vi "Flatten Value.vi"(0 "Path In":refnum<class "Path.lvclass">, 11 "Error In":errorcluster) -> (4 "Path Out":refnum<class "Path.lvclass">, 8 "Value":string, 15 "Error Out":errorcluster)   [LabVIEW 2016, in "Path.lvclass"]
uses:
  Path.lvclass
  Path.lvclass/Path.ctl
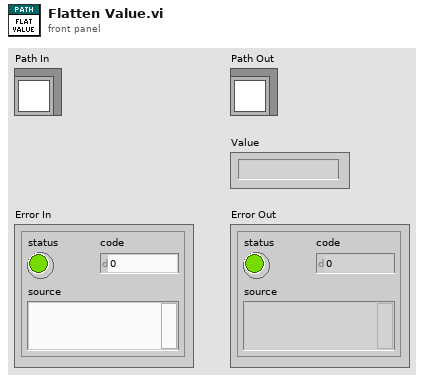
[diagram p1: front panel]
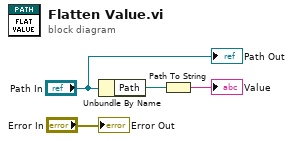
[diagram p0: block diagram]
diagram:
  n1 = Unbundle By Name("Path In") -> ("Path"=w4:path)
  n2 = Path To String(path=w4) -> (string=→"Value":string)
  "Path Out" <- "Path In"
  "Error Out" <- "Error In"
